vi "TSM SSC Digital Burst Pattern.vi"(0 "Digital TSM In":T1, 1 "Start Label":string, 2 "select digital function?":bool=TRUE caption="select digital function? (T)", 3 "wait until done?":bool=TRUE caption="wait until done? (T)", 7 "timeout (s)":dbl=10.0, 11 "error in":errorcluster) -> (4 "Digital TSM out":T1, 15 "error out":errorcluster)   [LabVIEW 2019]
doc: "Uses the start label you specify to burst the pattern on the pin(s) and pin group(s) you specify."
uses:
  TSM/TSM SSC Digital.ctl
  <vilib>/NI_TestStand_SemiconductorModule/NI_TestStand_Semiconductor_Module.lvlibp/PinMap/Digital Pattern/PinQueryContext/DigitalPatternPinQueryContext.lvclass
  SSC Digital/SSC Digital.ctl
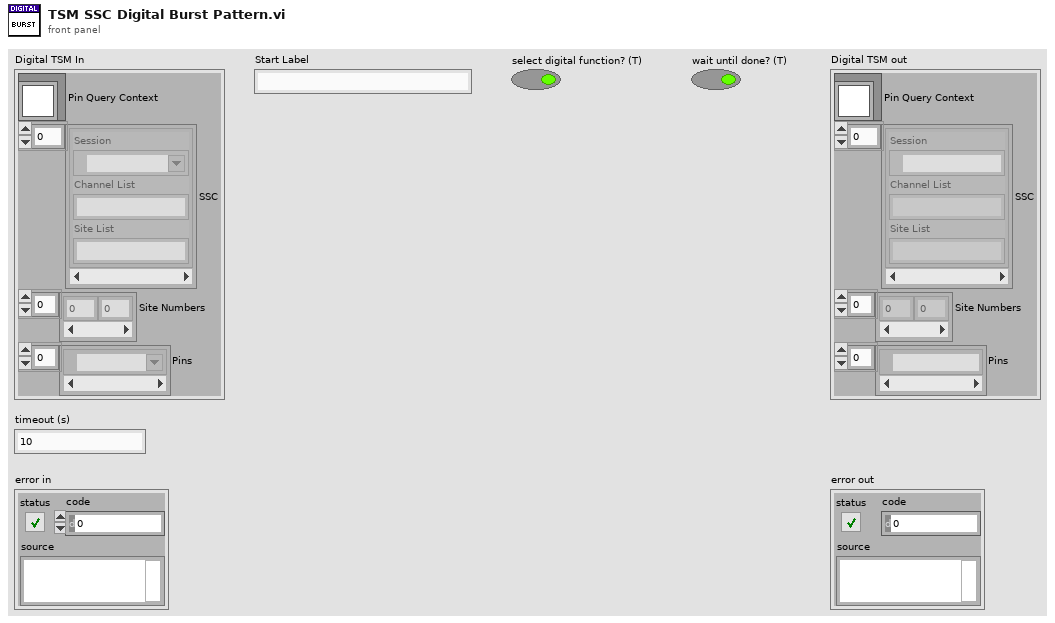
[diagram p1: front panel]
types:
  T1 = typedef "TSM SSC Digital.ctl" = cluster{"Pin Query Context":refnum<class "DigitalPatternPinQueryContext.lvclass">, "SSC":T2[], "Site Numbers":i32[], "Pins":tag[]}
  T2 = typedef "SSC Digital.ctl" = cluster{"Session":refnum<k15>, "Channel List":string, "Site List":string}
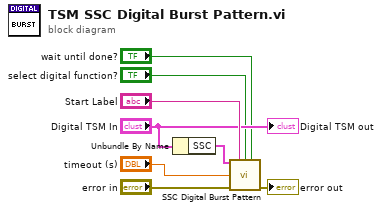
[diagram p0: block diagram]
diagram:
  n1 = Unbundle By Name("Digital TSM In") -> ("SSC"=w3:T2[])
  n2 = call "SSC Digital Burst Pattern.vi"("Digital SSC in"=w3, "Start Label"="Start Label", "select digital function?"="select digital function?", "wait until done?"="wait until done?", "timeout (s)"="timeout (s)", "error in"="error in") -> ("error out"=→"error out":errorcluster)  [unwired: 8 in, 1 out]
  "Digital TSM out" <- "Digital TSM In"
